vi "Do Scoring.vi"(11 "Submission LLB":path) -> (0 "error out":errorcluster, 2 "Test Summary":string, 3 "Score":T1)   [LabVIEW 2020, in "SOL-Scorer.lvlib"]
uses:
  SOL-Scorer.lvlib
  SoL Scoring/Score.ctl
  SoL Scoring/Score Entry.ctl
  SoL Scoring/SoL Scoring.lvlib
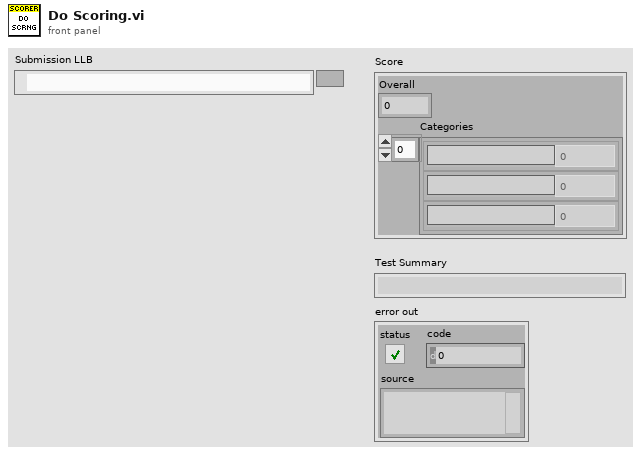
[diagram p1: front panel]
types:
  T1 = typedef "SoL Scoring.lvlib/Score.ctl" = cluster{"Overall":dbl, "Categories":T2[]}
  T2 = typedef "SoL Scoring.lvlib/Score Entry.ctl" = cluster{"Category":string, "Value":dbl}
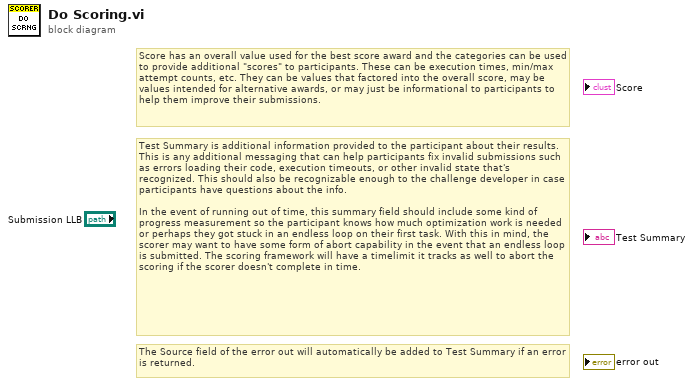
[diagram p0: block diagram]
diagram:
  # "The Source field of the error out will automatically be added to Test Summary if an error is returned."
  # "Test Summary is additional information provided to the participant about their results. This is any additional messaging that can help participants fix invalid submissions such as errors loading their code, execution timeouts, or other invalid state that's recognized. This should also be recognizable enough to the challenge developer in case participants have questions about the info.\n\nIn the event of running out of time, this summary field should include some kind of progress measurement so the participant knows how much optimization work is needed or perhaps they got stuck in an endless loop on their first task. With this in mind, the scorer may want to have some form of abort capability in the event that an endless loop is submitted. The scoring framework will have a timelimit it tracks as well to abort the scoring if the scorer doesn't complete in time."
  # "Score has an overall value used for the best score award and the categories can be used to provide additional \"scores\" to participants. These can be execution times, min/max attempt counts, etc. They can be values that factored into the overall score, may be values intended for alternative awards, or may just be informational to participants to help them improve their submissions."
